vi "Wiimote register for extension events.vi"(8 "error in":errorcluster, 11 "LV WiiMote Interface In":T1) -> (0 "error out":errorcluster, 3 "LV WiiMote Interface out":T1)   [LabVIEW 2012, in "LV Wiimote Interface.lvclass"]
uses:
  LV Wiimote Interface.lvclass
  Controls/LV Wiimote Interface.ctl
  LV Wiimote Interface.lvclass/LV Wiimote Interface.ctl
  Event Callback VIs/Wiimote Extension Changed Callback.vi
  C:/Program Files/National Instruments/LabVIEW 2012/vi.lib/LabVIEW Hacker/WiiMote/Dependencies/WiimoteLib.dll
  Program Files/National Instruments/LabVIEW 2012/vi.lib/LabVIEW Hacker/WiiMote/Dependencies/WiimoteLib.dll
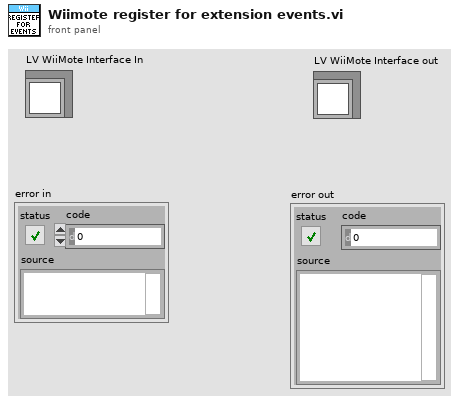
[diagram p1: front panel]
types:
  T1 = typedef "LV Wiimote Interface.ctl" = refnum<class "LV Wiimote Interface.lvclass">
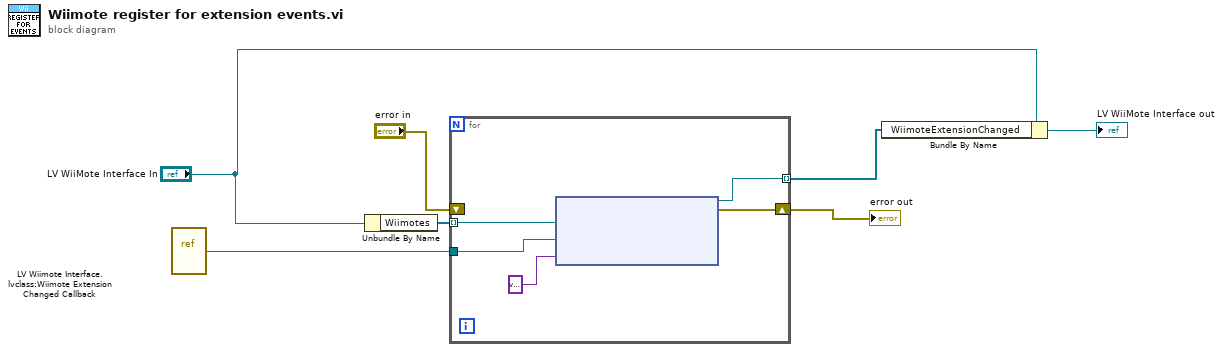
[diagram p0: block diagram]
diagram:
  n1 = vi-ref "LV Wiimote Interface.lvclass:Wiimote Extension Changed Callback.vi"() -> ("vi reference"=w4:refnum<vi>)
  n2 = Unbundle By Name("LV WiiMote Interface In") -> ("Wiimotes"=w7:refnum<k24>[])
  n3 = for {
    tunnel: w7 -> [w12] mode=indexing
    shift-right: [w11] -> w5
    shift-left: "error in" -> [_]
    tunnel: [w10] -> w2 mode=indexing
    tunnel: w4 -> [w9]
    n4 = node(w12, w9, variant ("User Parameter")) -> (w10:refnum<k27>, w11:errorcluster)  [unwired: 2 in]
  }
  "error out" <- w5
  n5 = Bundle By Name(cluster="LV WiiMote Interface In", "WiimoteExtensionChanged"=w2) -> (→"LV WiiMote Interface out":T1)
